vi "bitDepthToBytes.vi"(10 "bit depth":dbl=12.0) -> (3 "bytes":dbl=2.0)   [LabVIEW 2017]
uses:
  <vilib>/Analysis/1siggen.llb/Ramp Pattern by Samples.vi
  <vilib>/Analysis/NI_AALBase.lvlib
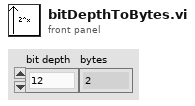
[diagram p1: front panel]
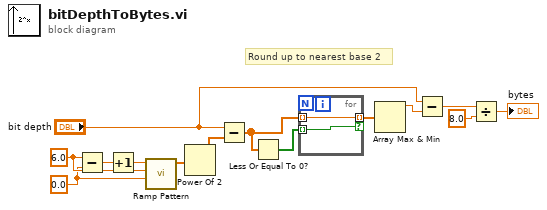
[diagram p0: block diagram]
diagram:
  w13 = 0.0 ("start")
  w14 = 6.0 ("end")
  # "Round up to nearest base 2"
  n1 = Subtract(x=w14, y=w13) -> (x-y=w12:dbl)
  n2 = Increment(x=w12) -> (x+1=w11:dbl)
  n3 = call-poly <vilib>:"Ramp Pattern.vi"("start"=w13, "end"=w14, "samples"=w11) -> ("Ramp Pattern"=w10:dbl[])  [unwired: 7 in, 1 out]
  n4 = Power Of 2(x=w10) -> (2^x=w3:dbl[])
  n5 = Subtract(x="bit depth", y=w3) -> (x-y=w8:dbl[])
  n6 = Less Or Equal To 0?(x=w8) -> (x <= 0?=w9:bool[])
  n7 = for {
    tunnel: w9 -> [w15] mode=indexing
    tunnel: w8 -> [w16] mode=indexing
    tunnel: [w16] -> w2 mode=indexing if=w15
  }
  n8 = Array Max & Min(array=w2) -> (max value=w7:dbl)  [unwired: 3 out]
  n9 = Subtract(x="bit depth", y=w7) -> (x-y=w6:dbl)
  n10 = Divide(x=w6, y=8.0) -> (x/y=→"bytes":dbl)
